vi "TPNT_SendAsyncStream.vi"(5 "logfile":path, 7 "notifier":refnum<notifier>, 9 "UTC":bool, 11 "Objects":T1[](array[typedef])) -> ()   [LabVIEW 2016]
uses:
  TPNT_Refnum.ctl
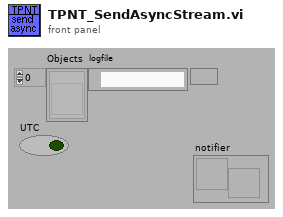
[diagram p1: front panel]
types:
  T1 = typedef "TPNT_Refnum.ctl" = refnum<vi>
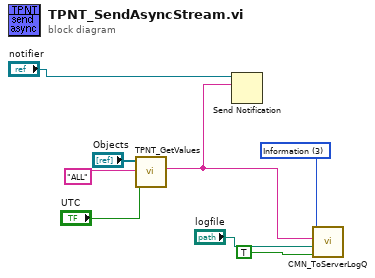
[diagram p0: block diagram]
diagram:
  w2 = u16 3 items=["command", "imediateReply", "Callback Reply", "Information", "none"] ("type")
  n1 = call "TPNT_GetValues.vi"("UTC"="UTC", "device"="ALL", "Objects"="Objects") -> ("full out"=w1:string)  [unwired: 8 out]
  n2 = Send Notification(notification=w1, notifier="notifier") -> ()  [unwired: 1 in, 2 out]
  n3 = call "CMN_ToServerLogQ.vi"("Log"=TRUE, "file"="logfile", "string"=w1, "type"=w2) -> ()  [unwired: 2 in, 5 out]
